vi "Keithley 6514 Math Config.vi"(0 "Resource In":refnum<visa-resource-name>, 1 "Check For SCPI Errors? (T)":bool=TRUE, 5 "calculation1 (Math OFF:2)":u16(ring)=2 items=["mx + b ON", "percent ON", "Math OFF"], 7 "slope (1)":dbl=1.0 min=-9.99999e+20 max=9.99999e+20 step=1.0 format="%.5e", 9 "y-intercept (0)":dbl min=-9.9999e+20 max=9.99999e+20 step=1.0 format="%.5e", 11 "error in (no error)":T1, 12 "percent ref value (1)":dbl=1.0 min=-9.99999e+20 max=9.99999e+20 step=1.0 format="%.5e", 13 "Math Units (\"MXB\")":string="MXB") -> (4 "Resource Out (dupl)":refnum<visa-resource-name>, 15 "error out":T1)   [LabVIEW 2009, in "Keithley 6514 LV 2009.lvlib"]
doc: "This VI is used to configure the setup for math calculation 1 which is either the mX + b or the percent calculation.\n\nTo read the results of the calculation, use the Math Read VI.\n\ncalculation1:\n0 = mX+b\n1 = Percent\n2 = Math Off\n\nMath Units:\nCan be up to three alphanumeric characters. \n\nslope:\n-9.99999e20 to +9.99999e20\n\noffset:\n-9.99999e20 to +9.99999e20\n\npercent target value:\n-9.99999e20 to +9.99999e20"
uses:
  Keithley 6514 LV 2009.lvlib
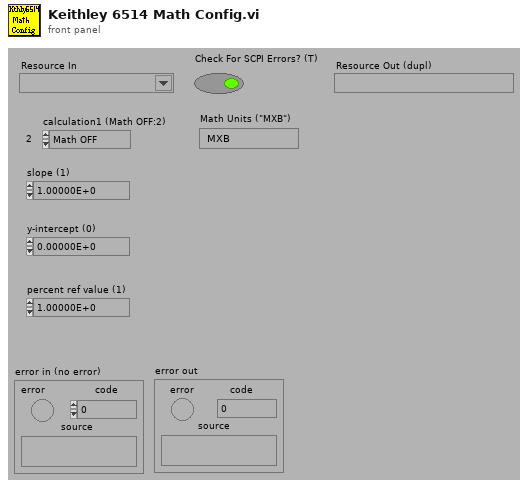
[diagram p1: front panel]
types:
  T1 = cluster{"error":bool, "code":i32, "source":string}
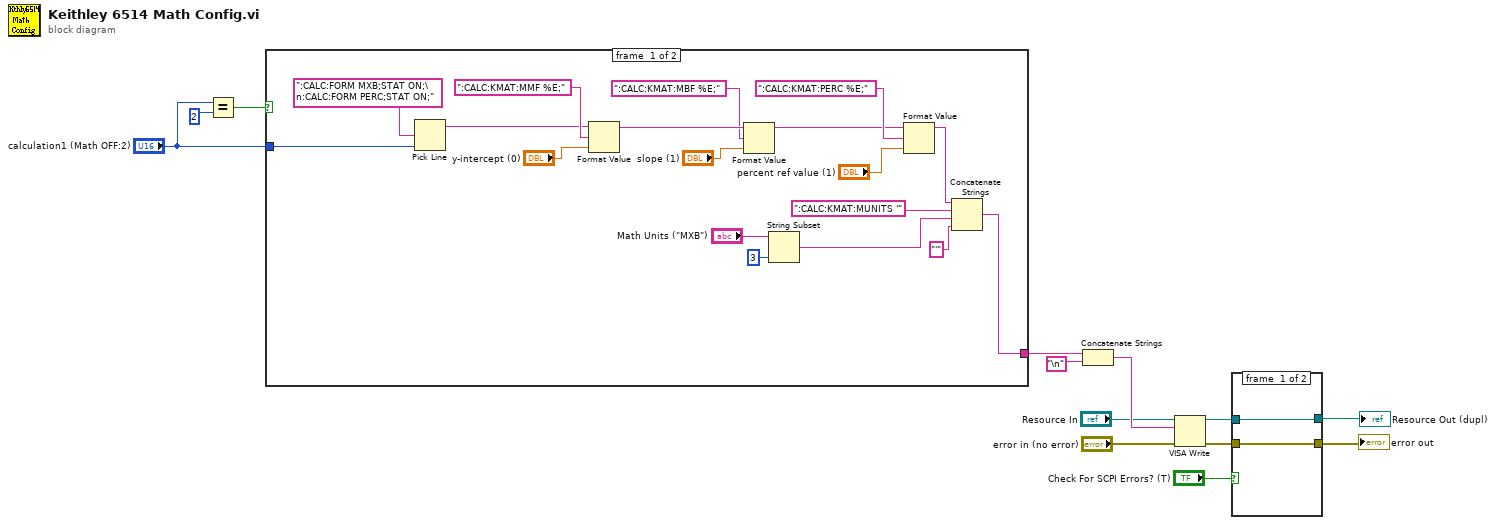
[diagram p0: block diagram]
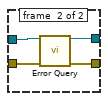
[diagram p2: hidden frame]
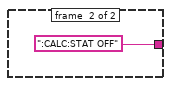
[diagram p3: hidden frame]
diagram:
  n1 = Equal?(x="calculation1 (Math OFF:2)", y=u16 2) -> (x = y?=w12:bool)
  n2 = case shown="True" w12 {
    tunnel: "calculation1 (Math OFF:2)" -> [w17 _]
    tunnel: [w16 ":CALC:STAT OFF"] -> w10
    frame #0 {
      n3 = Pick Line(multi-line string=":CALC:FORM MXB;STAT ON;\n:CALC:FORM PERC;STAT ON;", line index=w17) -> (output string=w20:string)  [unwired: 1 in]
      n4 = Format Value(string ("")=w20, format string=":CALC:KMAT:MMF %E;", value (0)="y-intercept (0)") -> (output string=w24:string)
      n5 = Format Value(string ("")=w24, format string=":CALC:KMAT:MBF %E;", value (0)="slope (1)") -> (output string=w25:string)
      n6 = String Subset(string="Math Units (\"MXB\")", length (rest)=3 ("length (rest)")) -> (substring=w15:string)  [unwired: 1 in]
      n7 = Format Value(string ("")=w25, format string=":CALC:KMAT:PERC %E;", value (0)="percent ref value (1)") -> (output string=w28:string)
      n8 = Concatenate Strings(w28, ":CALC:KMAT:MUNITS '", w15, "'") -> (w16:string)
    }
    frame #1 {
    }
  }
  n9 = Concatenate Strings(w10, "\n") -> (w8:string)
  n10 = VISA Write(VISA resource name="Resource In", write buffer=w8, error in (no error)="error in (no error)") -> (VISA resource name out=w4:refnum<visa-resource-name>, error out=w3:errorcluster)  [unwired: 1 out]
  n11 = case shown="True" "Check For SCPI Errors? (T)" {
    tunnel: w4 -> [w34 w38]
    tunnel: w3 -> [w33 w37]
    tunnel: [w34 w36] -> w2
    tunnel: [w33 w35] -> w1
    frame #0 {
    }
    frame #1 {
      n12 = call "Error Query.vi"("VISA Resource In"=w38, "error in (no error)"=w37) -> ("VISA Resource Out (dupl)"=w36:refnum<visa-resource-name>, "error out"=w35:errorcluster)  [unwired: 10 in, 2 out]
    }
  }
  "error out" <- w1
  "Resource Out (dupl)" <- w2
